vi "init runtime test.vi"() -> ()   [LabVIEW 2013, in "Profibus Module tests.lvlib"]
uses:
  Profibus Module tests.lvlib
  <vilib>/NI/Tag Bus/dictionary/data dictionary.lvclass
  execution/Profibus Module runtime.lvclass
  channel/Profibus channel.lvclass
panel:
  out "tags found":bool
  out "no error":errorcluster
  out "expected execution settings":bool
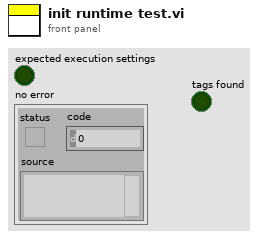
[diagram p1: front panel]
types:
  T1 = typedef "TBM channel.lvclass/data tables.ctl" = cluster{"input data":T2, "processing parameter":T2, "processing result":T2, "output data":T2}
  T2 = typedef "tag bus.lvlib/dictionary table pair.ctl" = cluster{"data dictionary":refnum<class "data dictionary.lvclass">, "data table":T3}
  T3 = typedef "tag bus.lvlib/data table.lvlib/data table.ctl" = cluster{"Double":dbl[], "Single":sgl[], "I64":i64[], "I32":i32[], "I16":i16[], "I8":i8[], "U64":u64[], "U32":u32[], "U16":u16[], "U8":u8[], "Boolean":bool[], "String":string[], "Array of Double":cluster{"DBL Array":dbl[]}[], "Array of Single":cluster{"SGL Array":sgl[]}[], "Array of I64":cluster{"I64 Array":i64[]}[], "Array of I32":cluster{"I32 Array":i32[]}[], "Array of I16":cluster{"I16 Array":i16[]}[], "Array of I8":cluster{"I8 Array":i8[]}[], "Array of U64":cluster{"U64 Array":u64[]}[], "Array of U32":cluster{"U32 Array":u32[]}[], "Array of U16":cluster{"U16 Array":u16[]}[], "Array of U8":cluster{"U8 Array":u8[]}[], "Array of Boolean":cluster{"Boolean Array":bool[]}[], "Array of String":cluster{"String Array":string[]}[]}
  T4 = typedef "TBM module execution interface.lvclass/execution settings.ctl" = cluster{"reads inputs":bool, "processes data":bool, "writes outputs":bool}
  T5 = typedef "tag bus.lvlib/tag descriptor.lvclass/Data Type.ctl" = enum16{"Double", "Single", "I64", "I32", "I16", "I8", "U64", "U32", "U16", "U8", "Boolean", "String", "Array of Double", "Array of Single", "Array of I64", "Array of I32", "Array of I16", "Array of I8", "Array of U64", "Array of U32", "Array of U16", "Array of U8", "Array of Boolean", "Array of String"}
  T6 = typedef "TBM channel.lvclass/channel classification.ctl" = enum16{"input data", "output data", "processing parameter", "processing result"}
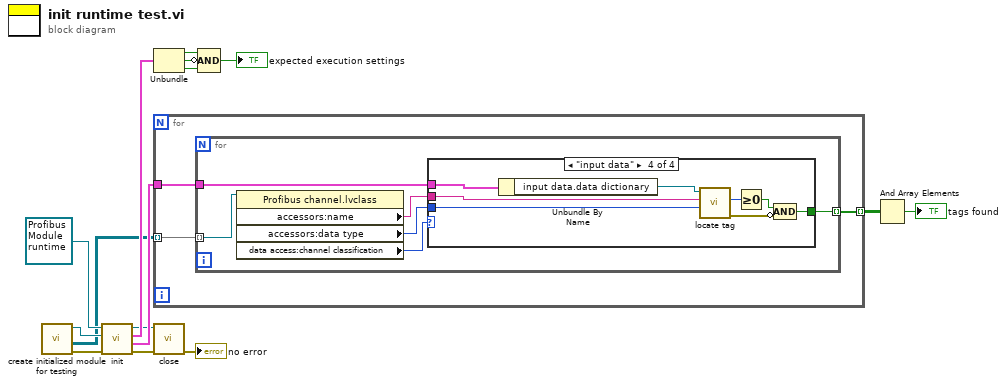
[diagram p0: block diagram]
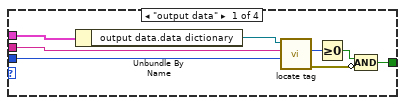
[diagram p2: hidden frame]
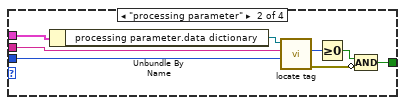
[diagram p3: hidden frame]
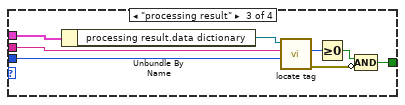
[diagram p4: hidden frame]
diagram:
  n1 = call "create initialized module for testing.vi"() -> ("error out"=w2:errorcluster, "2d channels"=w1:refnum<class "Profibus channel.lvclass">[][], "Profibus Module configuration out"=w3:refnum<class "Profibus Module configuration.lvclass">)  [unwired: 6 in, 3 out]
  n2 = call-dynamic "init.vi"("error in"=w2, "TBM module configuration in"=w3, "Profibus Module runtime in"=refnum<class "Profibus Module runtime.lvclass"> refnum ("tag bus configurable plugin module")) -> ("error out"=w7:errorcluster, "data allocations"=w15:T1, "execution settings"=w14:T4, "Profibus Module runtime out"=w6:refnum<class "Profibus Module runtime.lvclass">)  [unwired: 5 in]
  n3 = Unbundle(w14) -> ("reads inputs"=w13:bool, "processes data"=w11:bool, "writes outputs"=w12:bool)
  n4 = for {
    tunnel: w15 -> [w18]
    tunnel: w1 -> [w17] mode=indexing
    tunnel: [w16] -> w9 mode=indexing
    n5 = for {
      tunnel: w18 -> [w22]
      tunnel: w17 -> [w24] mode=indexing
      tunnel: [w19] -> w16 mode=indexing
      n6 = property class="Profibus channel.lvclass"(reference=w24) -> ("accessors:name"=w20:string, "accessors:data type"=w21:T5, "data access:channel classification"=w23:T6)  [unwired: 1 in, 2 out]
      n7 = case shown="\"input data\"" w23 {
        tunnel: w22 -> [w32 w40 w48 w56]
        tunnel: w21 -> [w30 w38 w46 w54]
        tunnel: w20 -> [w29 w37 w45 w53]
        tunnel: [w25 w33 w41 w49] -> w19
        frame "output data" {
          n8 = Unbundle By Name(w32) -> ("output data.data dictionary"=w31:refnum<class "data dictionary.lvclass">)
          n9 = call <vilib>:"locate tag.vi"("data type"=w30, "name"=w29, "data dictionary in"=w31) -> ("error out"=w26:errorcluster, "index"=w28:i32)  [unwired: 6 in, 1 out]
          n10 = Greater Or Equal To 0?(x=w28) -> (x >= 0?=w27:bool)
          n11 = Compound Arithmetic op=AND(w27, invert w26) -> (w25:bool)
        }
        frame "processing parameter" {
          n12 = Unbundle By Name(w40) -> ("processing parameter.data dictionary"=w39:refnum<class "data dictionary.lvclass">)
          n13 = call <vilib>:"locate tag.vi"("data type"=w38, "name"=w37, "data dictionary in"=w39) -> ("error out"=w34:errorcluster, "index"=w36:i32)  [unwired: 6 in, 1 out]
          n14 = Greater Or Equal To 0?(x=w36) -> (x >= 0?=w35:bool)
          n15 = Compound Arithmetic op=AND(w35, invert w34) -> (w33:bool)
        }
        frame "processing result" {
          n16 = Unbundle By Name(w48) -> ("processing result.data dictionary"=w47:refnum<class "data dictionary.lvclass">)
          n17 = call <vilib>:"locate tag.vi"("data type"=w46, "name"=w45, "data dictionary in"=w47) -> ("error out"=w42:errorcluster, "index"=w44:i32)  [unwired: 6 in, 1 out]
          n18 = Greater Or Equal To 0?(x=w44) -> (x >= 0?=w43:bool)
          n19 = Compound Arithmetic op=AND(w43, invert w42) -> (w41:bool)
        }
        frame "input data" {
          n20 = Unbundle By Name(w56) -> ("input data.data dictionary"=w55:refnum<class "data dictionary.lvclass">)
          n21 = call <vilib>:"locate tag.vi"("data type"=w54, "name"=w53, "data dictionary in"=w55) -> ("error out"=w50:errorcluster, "index"=w52:i32)  [unwired: 6 in, 1 out]
          n22 = Greater Or Equal To 0?(x=w52) -> (x >= 0?=w51:bool)
          n23 = Compound Arithmetic op=AND(w51, invert w50) -> (w49:bool)
        }
      }
    }
  }
  n24 = call-dynamic "close.vi"("error in"=w7, "Profibus Module runtime in"=w6) -> ("error out"=→"no error":errorcluster)  [unwired: 9 in]
  n25 = Compound Arithmetic op=AND(w13, invert w11, w12) -> (→"expected execution settings":bool)
  n26 = And Array Elements(Boolean array=w9) -> (logical AND=→"tags found":bool)
